vi "Test - Serial.vi"() -> ()   [LabVIEW 2013]
panel:
  out "VISA port":refnum<visa-resource-name>
  out "error out":errorcluster
  out "VISA Port":refnum<visa-resource-name>="COM4"
  out "#Bytes (Pairing)":u32
  in  "Frequency":u8(ring)=1 items=["CHAN0", "CHAN1", "CHAN2", "CHAN3", "CHAN4", "CHAN5"]
  in  "Threshold":u16=2047
  out "Readback":u8[](array[numeric])
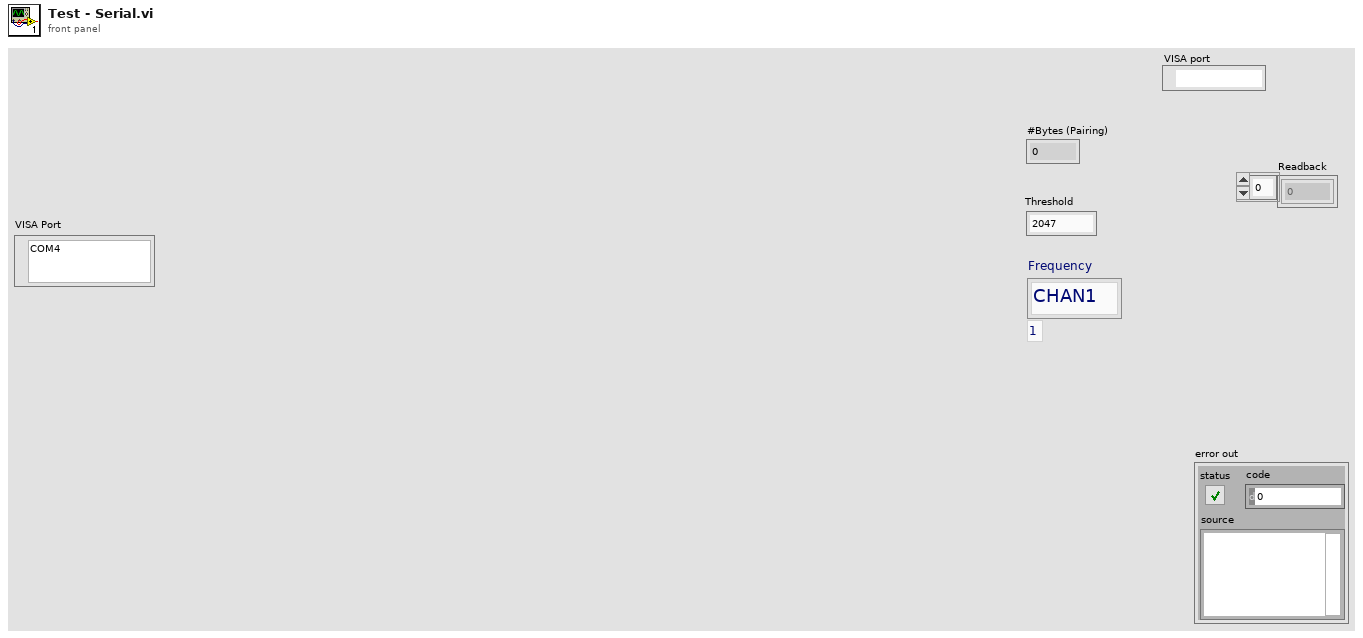
[diagram p1: front panel]
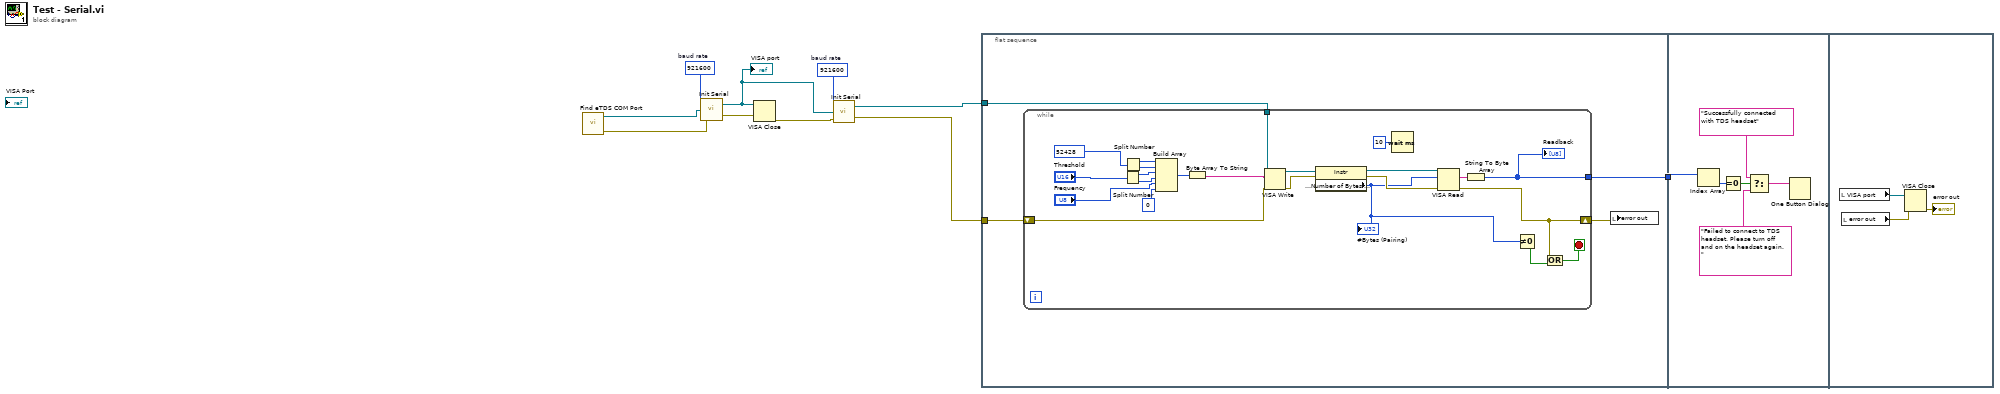
[diagram p0: block diagram]
diagram:
  w5 = u32 921600  # baud rate
  w10 = u32 921600  # baud rate
  n1 = call "Find eTDS COM Port.vi"() -> ("USB port"=w9:refnum<visa-resource-name>, "error out"=w8:errorcluster)  [unwired: 1 in, 1 out]
  n2 = call "Init Serial.vi"("error in (no error)"=w8, "VISA resource name"=w9, "baud rate"=w10) -> ("error out"=w6:errorcluster, "VISA resource name out"=w3:refnum<visa-resource-name>)
  "VISA port" <- w3
  n3 = VISA Close(VISA resource name=w3, error in (no error)=w6) -> (error out=w4:errorcluster)
  n4 = call "Init Serial.vi"("error in (no error)"=w4, "VISA resource name"=w3, "baud rate"=w5) -> ("error out"=w1:errorcluster, "VISA resource name out"=w2:refnum<visa-resource-name>)
  n5 = flat-sequence {
    tunnel: w2 -> [w14]
    tunnel: w1 -> [w13]
    tunnel: [w12] -> w7
    tunnel: w7 -> [w38]
    frame #0 {
      n6 = while {
        tunnel: w14 -> [w22]
        shift-right: [w18] -> w11
        shift-left: w13 -> [w21]
        tunnel: [w15] -> w12
        stop <- w16 stop-if-true
        n7 = Split Number(x="Threshold") -> (hi(x)=w36:u8, lo(x)=w37:u8)
        n8 = Split Number(x=u16 52428 ("ChnA")) -> (hi(x)=w35:u8, lo(x)=w34:u8)
        n9 = Build Array(w35, w34, w36, w37, "Frequency", u8 0 ("ChnA")) -> (w33:u8[])
        n10 = Byte Array To String(unsigned byte array=w33) -> (string=w29:string)
        n11 = VISA Write(VISA resource name=w22, write buffer=w29, error in (no error)=w21) -> (VISA resource name out=w28:refnum<visa-resource-name>, error out=w27:errorcluster)  [unwired: 1 out]
        n12 = property class="Instr"(reference=w28, error in=w27) -> (reference out=w25:refnum<visa-resource-name>, error out=w24:errorcluster, "Serial Settings:Number of Bytes at Serial Port"=w19:u32)
        "#Bytes (Pairing)" <- w19
        n13 = Wait (ms)(milliseconds to wait=u32 10) -> ()  [unwired: 1 out]
        n14 = VISA Read(VISA resource name=w25, byte count=w19, error in (no error)=w24) -> (read buffer=w23:string, error out=w18:errorcluster)  [unwired: 2 out]
        n15 = String To Byte Array(string=w23) -> (unsigned byte array=w15:u8[])
        "Readback" <- w15
        n16 = Not Equal To 0?(x=w19) -> (x != 0?=w17:bool)
        n17 = Or(x=w18, y=w17) -> (x .or. y?=w16:bool)
      }
      n18 = local write "error out"(w11) -> ()
    }
    frame #1 {
      n19 = Index Array "Index Array"(array=w38) -> (element=w42:u8)  [unwired: 1 in]
      n20 = Equal To 0?(x=w42) -> (x = 0?=w43:bool)
      n21 = Select(t="Successfully connected with TDS headset", s=w43, f="Failed to connect to TDS headset. Please turn off and on the headset again.") -> (s? t:f=w39:string)
      n22 = One Button Dialog(message=w39) -> ()  [unwired: 1 in, 1 out]
    }
    frame #2 {
      n23 = local read "VISA port"() -> (w45:refnum<visa-resource-name>)
      n24 = local read "error out"() -> (w44:errorcluster)
      n25 = VISA Close(VISA resource name=w45, error in (no error)=w44) -> (error out=→"error out":errorcluster)
    }
  }
